vi "Configure Protection.vi"(6 "Protection (None)":T1, 8 "error in (no error)":errorcluster, 10 "Limit":dbl, 11 "GEN40-38-LAN in":refnum<class "GEN40-38-LAN.lvclass">) -> (0 "error out":errorcluster, 3 "GEN40-38-LAN out":refnum<class "GEN40-38-LAN.lvclass">)   [LabVIEW 2018, in "GEN40-38-LAN.lvlib" / "GEN40-38-LAN.lvclass"]
doc: "Configure Protection setting, available options:\n\n0: None\n1: Over Voltage\n2: Under Voltage\n3: Over Current\n\nDbl Precision Limit"
uses:
  GEN40-38-LAN.lvclass
  PPLs/Power Supply/Parent/Power_Supply.lvlibp/Custom Control/Protection.ctl
  PPLs/Power Supply/Parent/Power_Supply.lvlibp/Power Supply.lvclass
  C:/Projects/LabVIEW/PPLs/Power Supply/Parent/Power_Supply.lvlibp/Power Supply.lvclass
  PPLs/Power Supply/Parent/Power_Supply.lvlibp
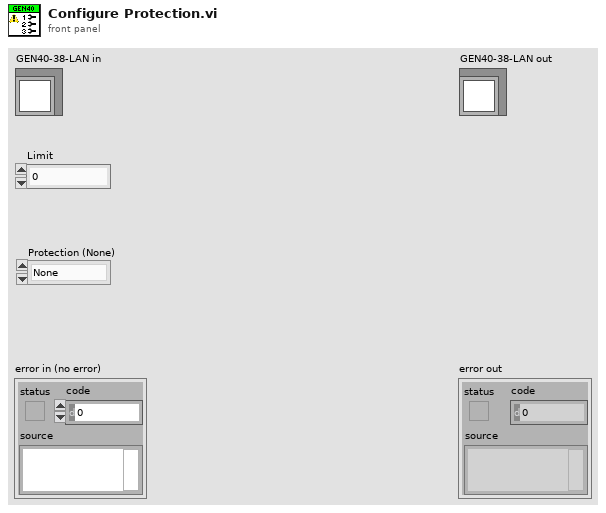
[diagram p1: front panel]
types:
  T1 = typedef "Power_Supply.lvlibp/Protection.ctl" = enum16{"None", "Over Volt", "Under Volt", "Over Current"}
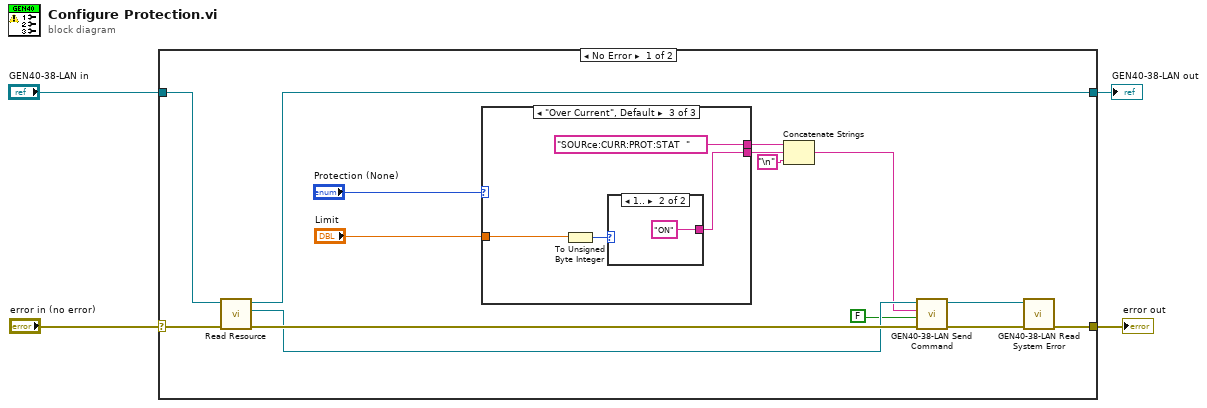
[diagram p0: block diagram]
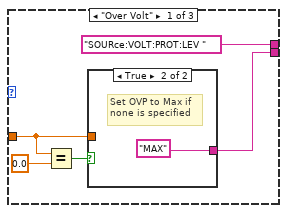
[diagram p2: hidden frame]
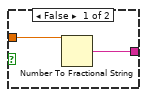
[diagram p3: hidden frame]
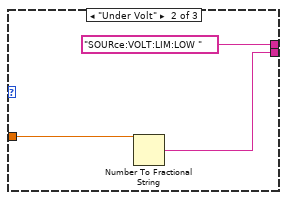
[diagram p4: hidden frame]
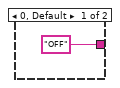
[diagram p5: hidden frame]
diagram:
  n1 = case shown="No Error" "error in (no error)" {
    selector: "error in (no error)" -> [w19 w38]
    tunnel: [w17 w38] -> w3
    tunnel: [w13 w37] -> w2
    tunnel: "GEN40-38-LAN in" -> [w18 w37]
    frame No Error {
      n2 = call "Read Resource.vi"("error in"=w19, "Power Supply in"=w18) -> ("error out"=w14:errorcluster, "Resource"=w12:refnum<visa-resource-name>, "Power Supply out"=w13:refnum<class "GEN40-38-LAN.lvclass">)  [unwired: 7 in]
      n3 = case shown="\"Over Current\", Default" "Protection (None)" {
        tunnel: ["SOURce:VOLT:PROT:LEV " "SOURce:VOLT:LIM:LOW " "SOURce:CURR:PROT:STAT  "] -> w10
        tunnel: "Limit" -> [w21 w29 w33]
        tunnel: [w20 w28 w31] -> w8
        frame "Over Volt" {
          n4 = Equal?(x=w21, y=0.0) -> (x = y?=w22:bool)
          n5 = case shown="True" w22 {
            tunnel: [w25 "MAX"] -> w20
            tunnel: w21 -> [w26 _]
            frame False {
              n6 = Number To Fractional String(number=w26) -> (F-format string=w25:string)  [unwired: 3 in]
            }
            frame True {
              # "Set OVP to Max if\nnone is specified"
            }
          }
        }
        frame "Under Volt" {
          n7 = Number To Fractional String(number=w29) -> (F-format string=w28:string)  [unwired: 3 in]
        }
        frame "Over Current", Default {
          n8 = To Unsigned Byte Integer(number=w33) -> (unsigned 8bit integer=w32:u8)
          n9 = case shown="1.." w32 {
            tunnel: ["OFF" "ON"] -> w31
            frame 0, Default {
            }
            frame 1.. {
            }
          }
        }
      }
      n10 = Concatenate Strings(w10, w8, "\n" ("string")) -> (w6:string)
      n11 = call "GEN40-38-LAN Send Command.vi"("error in (no error)"=w14, "Wait for Response?"=FALSE, "Command"=w6, "VISA resource name"=w12) -> ("error out"=w16:errorcluster, "VISA resource name out"=w15:refnum<visa-resource-name>)  [unwired: 5 in, 1 out]
      n12 = call "GEN40-38-LAN Read System Error.vi"("error in (no error)"=w16, "Resource"=w15) -> ("error out"=w17:errorcluster)  [unwired: 9 in]
    }
    frame Error {
    }
  }
  "error out" <- w3
  "GEN40-38-LAN out" <- w2
